vi "common_global_app_event_fgv.vi"(7 "action (0: get)":enum16{"get", "init"}(ring), 8 "error in (no error)":errorcluster) -> (0 "error out":errorcluster, 3 "app event":refnum<user-event>)   [LabVIEW 2019]
doc: "Used to initialize this app to use the framework. Also used to retrieve the event handle to connect new modules to the framework. State \"init\" must be used before attempting to have modules on the framework talk to each other."
uses:
  common data types/common_event_data.ctl
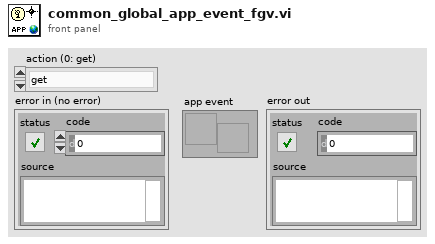
[diagram p1: front panel]
types:
  T1 = typedef "common_event_data.ctl" = cluster{"sender":string, "target":string, "msg":string, "data":variant}
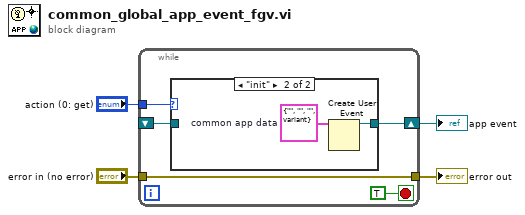
[diagram p0: block diagram]
diagram:
  n1 = while {
    shift-right: [w9] -> w1
    shift-left: _ -> [w6]
    tunnel: "action (0: get)" -> [w7]
    tunnel: "error in (no error)" -> [w5]
    tunnel: [w5] -> w2
    stop <- TRUE stop-if-true
    n2 = case shown="\"init\"" w7 {
      tunnel: [w10 w11] -> w9
      tunnel: w6 -> [w10 _]
      frame "get", Default {
      }
      frame "init" {
        w12 = T1 {"sender"="", "target"="", "msg"="", "data"=variant}  # common app data
        n3 = Create User Event(user event datatype=w12) -> (user event=w11:refnum<user-event>)  [unwired: 1 in, 1 out]
      }
    }
  }
  "app event" <- w1
  "error out" <- w2
